vi "Get Field.vi"(8 "error in (no error)":errorcluster, 11 "Instrument.1820 in":refnum<class "Instrument.OxfordVRM.lvclass">) -> (0 "error out":errorcluster, 2 "Field (T)":dbl, 3 "Instrument.1820 in":refnum<class "Instrument.OxfordVRM.lvclass">)   [LabVIEW 2016, in "Instrument.OxfordVRM.lvclass"]
uses:
  Instrument.OxfordVRM.lvclass
  Typedefs/Instrument.Oxford1820.Commands-enum.ctl
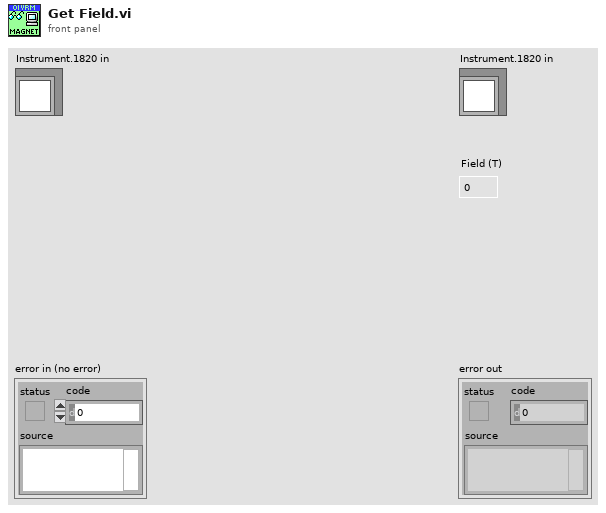
[diagram p1: front panel]
types:
  T1 = typedef "Instrument.OxfordVRM.lvclass/Instrument.Oxford1820.Commands-enum.ctl" = enum16{"setAction", "setTarget", "setSwitchHeat", "setLambda", "setFillMode", "setNeedleValve", "setMagnetField", "getStatus", "getTarget", "getSwitchHeat", "getPSUField", "newcommand", "getMagnetField"}
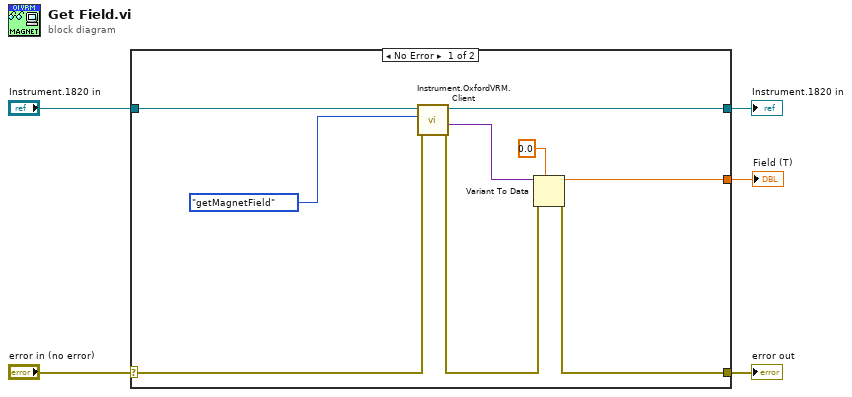
[diagram p0: block diagram]
diagram:
  n1 = case shown="No Error" "error in (no error)" {
    selector: "error in (no error)" -> [w13 w16]
    tunnel: [w9 w16] -> w4
    tunnel: "Instrument.1820 in" -> [w7 w15]
    tunnel: [w8 _] -> w2
    tunnel: [w6 w15] -> w1
    frame No Error {
      n2 = call "Instrument.OxfordVRM.Client.vi"("error in (no error)"=w13, "Commands"=Instrument.Oxford1820.Commands-enum."getMagnetField", "Instrument.1820 in"=w7) -> ("error out"=w10:errorcluster, "Data out"=w12:variant, "Instrument.1820 out"=w6:refnum<class "Instrument.OxfordVRM.lvclass">)  [unwired: 6 in]
      n3 = Variant To Data(error in=w10, type=0.0, Variant=w12) -> (data=w8:dbl, error out=w9:errorcluster)
    }
    frame Error {
    }
  }
  "error out" <- w4
  "Instrument.1820 in" <- w1
  "Field (T)" <- w2
